vi "validate.vi"(8 "error in":errorcluster, 11 "TEC configuration in":refnum<class "TEC configuration.lvclass">) -> (0 "error out":errorcluster, 3 "TEC configuration out":refnum<class "TEC configuration.lvclass">)   [LabVIEW 2013, in "TEC configuration.lvclass"]
doc: "This function performs validation of the configuration. This function should be safe to call at any point and should not rely on anything in the runtime environment."
uses:
  TEC configuration.lvclass
  <vilib>/NI/Tag Bus Module Framework/module configuration/TBM module configuration.lvclass
  TEC configuration.lvclass/TEC configuration.ctl
  <vilib>/NI/Configuration Framework/NISE_CEF_TreeControl.lvlib
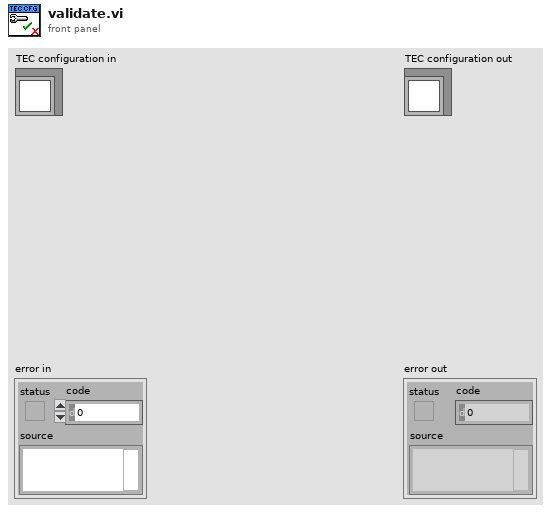
[diagram p1: front panel]
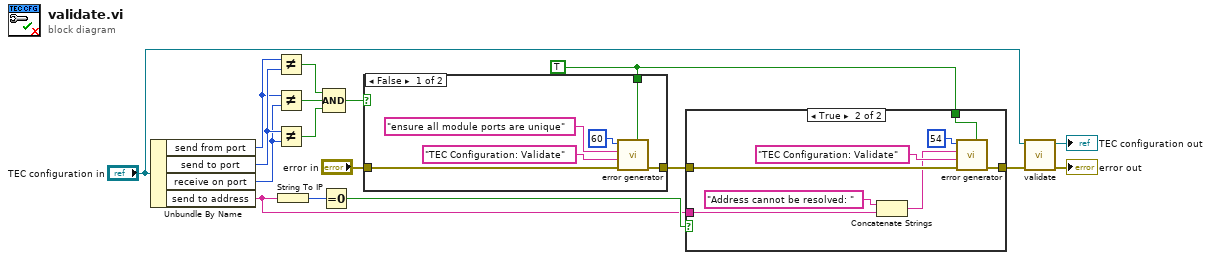
[diagram p0: block diagram]
diagram:
  w1 = TRUE ("concatenate (F)")
  n1 = Unbundle By Name("TEC configuration in") -> ("send from port"=w13:u16, "send to port"=w14:u16, "receive on port"=w12:u16, "send to address"=w2:string)
  n2 = Not Equal?(x=w13, y=w14) -> (x != y?=w11:bool)
  n3 = Not Equal?(x=w13, y=w12) -> (x != y?=w10:bool)
  n4 = Not Equal?(x=w14, y=w12) -> (x != y?=w9:bool)
  n5 = String To IP(1:w2) -> (0:w4:u32)
  n6 = Equal To 0?(x=w4) -> (x = 0?=w3:bool)
  n7 = Compound Arithmetic op=AND(w11, w10, w9) -> (w8:bool)
  n8 = case shown="False" w8 {
    tunnel: [w22 w24] -> w6
    tunnel: "error in" -> [w23 w24]
    tunnel: w1 -> [w18 _]
    frame False {
      n9 = call <vilib>:"error generator.vi"("concatenate (F)"=w18, "error in"=w23, "source"="TEC Configuration: Validate", "append error message"="ensure all module ports are unique", "error code (0)"=60) -> ("error out"=w22:errorcluster)  [unwired: 4 in]
    }
    frame True {
    }
  }
  n10 = case shown="True" w3 {
    tunnel: [w25 w32] -> w5
    tunnel: w6 -> [w25 w33]
    tunnel: w2 -> [_ w28]
    tunnel: w1 -> [_ w26]
    frame False {
    }
    frame True {
      n11 = Concatenate Strings("Address cannot be resolved: " ("string"), w28) -> (w27:string)
      n12 = call <vilib>:"error generator.vi"("concatenate (F)"=w26, "error in"=w33, "source"="TEC Configuration: Validate", "append error message"=w27, "error code (0)"=54) -> ("error out"=w32:errorcluster)  [unwired: 4 in]
    }
  }
  n13 = call-parent "validate.vi"("error in"=w5, "configuration in"="TEC configuration in") -> ("error out"=→"error out":errorcluster, "configuration out"=→"TEC configuration out":refnum<class "TEC configuration.lvclass">)  [unwired: 8 in]
